vi "Get Library Path.vi"() -> (3 "library path":path)   [LabVIEW 2020, in "libpcaplv.lvlib"]
uses:
  libpcaplv.lvlib
  <vilib>/Utility/sysdir.llb/System Directory Type.ctl
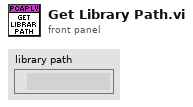
[diagram p1: front panel]
types:
  T1 = typedef "System Directory Type.ctl" = i32
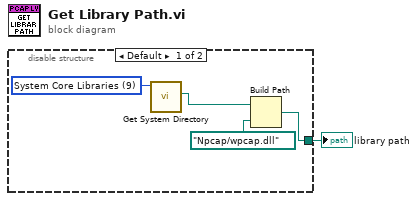
[diagram p0: block diagram]
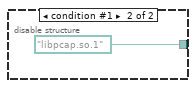
[diagram p2: hidden frame]
diagram:
  n1 = disable-structure shown="Default" {
    disable-tunnel: [w3 path "libpcap.so.1"] -> w1
    frame condition #0 (active) {
      w2 = T1 9 items=["User Home"=0, "User Desktop"=1, "User Documents"=2, "User Application Data"=3, "User Preferences"=4, "User Temporary"=5, "Public Documents"=6, "Public Application Data"=7, "Public Preferences"=8, "Public Cache"=13, "System Core Libraries"=9, "System Installed Libraries"=10, "Application Files"=11, "Boot Volume Root"=12] ("system directory type")
      n2 = call <vilib>:"Get System Directory.vi"("system directory type"=w2) -> ("system directory"=w5:path)  [unwired: 10 in]
      n3 = Build Path(base path=w5, name or relative path=path "Npcap/wpcap.dll") -> (appended path=w3:path)
    }
    frame condition #1 {
    }
  }
  "library path" <- w1
